vi "from string.vi"(8 "error in":errorcluster, 9 "data":string, 10 "version":string, 11 "TDMS datalogger configuration in":refnum<class "TDMS datalogger configuration.lvclass">) -> (0 "error out":errorcluster, 3 "TDMS datalogger configuration out":refnum<class "TDMS datalogger configuration.lvclass">)   [LabVIEW 2015, in "TDMS datalogger configuration.lvclass"]
doc: "Provides an interface for loading a module configuration from a file or other serialized data source. It is recommended that all children of this class store data in two sets--data required for its own initialization, and any data required for parent initialization--and that each implementation uses the <b>Call Parent Method</b> primitive to de-serialize parent information. As a result, it is expected that every module configuration class calls <b>component configuration.lvclass:From String.vi</b>."
uses:
  TDMS datalogger configuration.lvclass
  <vilib>/NI/Tag Bus Module Framework/channel/TBM channel.lvclass
  <vilib>/NI/LogRotate/options.ctl
  TDMS datalogger configuration.lvclass/TDMS datalogger configuration.ctl
  <vilib>/NI/Tag Bus Module Framework/module configuration/TBM module configuration.lvclass
  <vilib>/NI/Configuration Framework/serializable configuration/NISE_CEF_serializable configuration.lvclass
  <vilib>/NI/LogRotate/LogRotate.lvclass
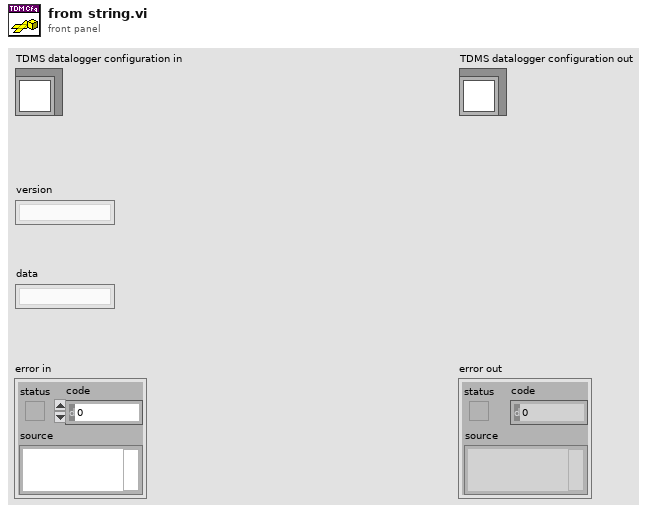
[diagram p1: front panel]
types:
  T1 = cluster{"channel":refnum<class "TBM channel.lvclass">}[]
  T2 = typedef "LogRotate.lvclass/options.ctl" = cluster{"max file size (bytes)":i64, "rotate count":u32, "max age (days)":dbl, "No archive dir":bool, "Archive dir":path}
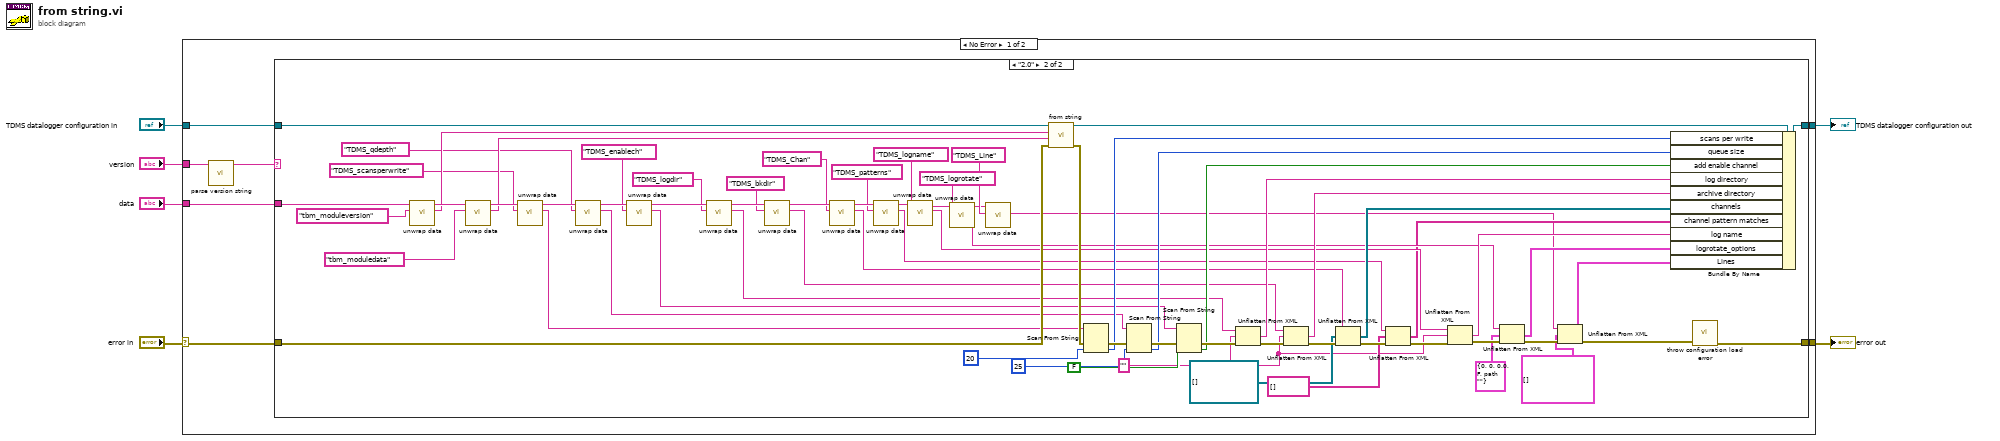
[diagram p0: block diagram]
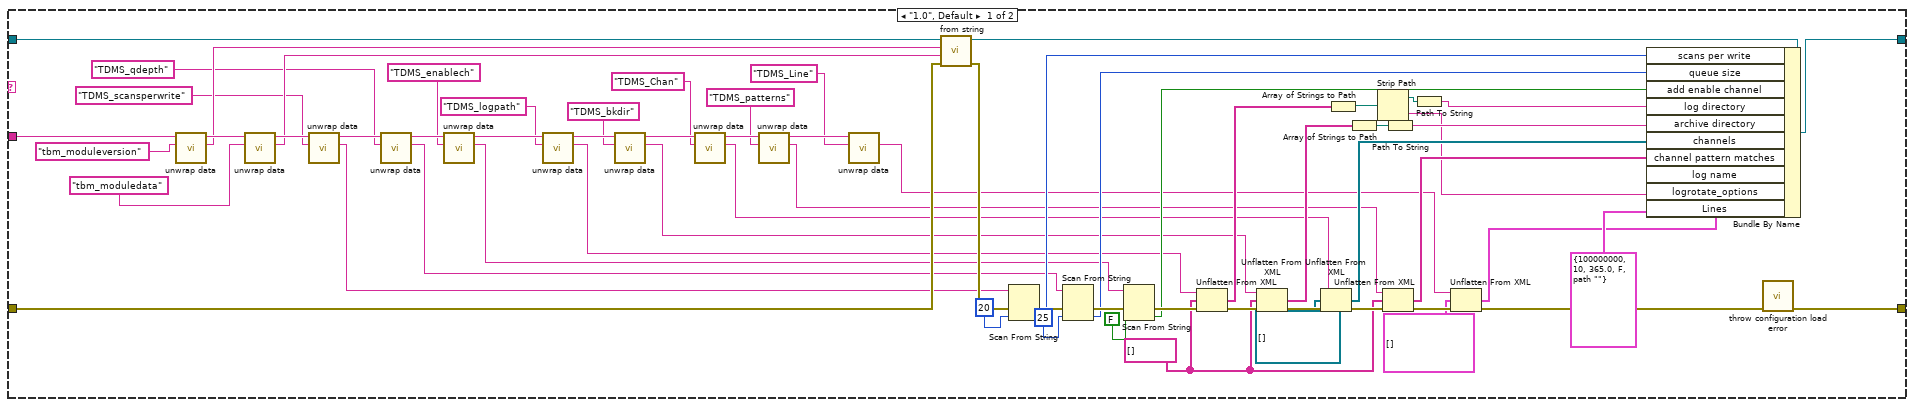
[diagram p2: hidden frame]
diagram:
  n1 = case shown="No Error" "error in" {
    selector: "error in" -> [w7 w150]
    tunnel: "data" -> [w13 _]
    tunnel: "TDMS datalogger configuration in" -> [w12 w149]
    tunnel: [w11 w149] -> w5
    tunnel: [w10 w150] -> w4
    tunnel: "version" -> [w9 _]
    frame No Error {
      n2 = call <vilib>:"parse version string.vi"("full version"=w9) -> ("major.minor version"=w8:string)  [unwired: 7 in, 3 out]
      n3 = case shown="\"2.0\"" w8 {
        tunnel: w13 -> [w61 w131]
        tunnel: w7 -> [w75 w145]
        tunnel: w12 -> [w78 w148]
        tunnel: [w77 w147] -> w11
        tunnel: [w34 w104] -> w10
        frame "1.0", Default {
          w30 = string[] [] ("array of strings")
          n4 = call <vilib>:"unwrap data.vi"("identifier"="tbm_moduleversion" ("additional identifier"), "data to unwrap"=w61) -> ("unwrapped data"=w60:string, "remaining string"=w67:string)  [unwired: 8 in]
          n5 = call <vilib>:"unwrap data.vi"("identifier"="tbm_moduledata" ("additional identifier"), "data to unwrap"=w67) -> ("unwrapped data"=w59:string, "remaining string"=w64:string)  [unwired: 8 in]
          n6 = call <vilib>:"unwrap data.vi"("identifier"="TDMS_scansperwrite" ("additional identifier"), "data to unwrap"=w64) -> ("unwrapped data"=w45:string, "remaining string"=w63:string)  [unwired: 8 in]
          n7 = call <vilib>:"unwrap data.vi"("identifier"="TDMS_qdepth" ("additional identifier"), "data to unwrap"=w63) -> ("unwrapped data"=w43:string, "remaining string"=w62:string)  [unwired: 8 in]
          n8 = call <vilib>:"unwrap data.vi"("identifier"="TDMS_enablech" ("additional identifier"), "data to unwrap"=w62) -> ("unwrapped data"=w41:string, "remaining string"=w49:string)  [unwired: 8 in]
          n9 = call <vilib>:"unwrap data.vi"("identifier"="TDMS_logpath" ("additional identifier"), "data to unwrap"=w49) -> ("unwrapped data"=w39:string, "remaining string"=w48:string)  [unwired: 8 in]
          n10 = call <vilib>:"unwrap data.vi"("identifier"="TDMS_bkdir" ("additional identifier"), "data to unwrap"=w48) -> ("unwrapped data"=w38:string, "remaining string"=w47:string)  [unwired: 8 in]
          n11 = call <vilib>:"unwrap data.vi"("identifier"="TDMS_Chan" ("additional identifier"), "data to unwrap"=w47) -> ("unwrapped data"=w37:string, "remaining string"=w33:string)  [unwired: 8 in]
          n12 = call <vilib>:"unwrap data.vi"("identifier"="TDMS_patterns", "data to unwrap"=w33) -> ("unwrapped data"=w29:string, "remaining string"=w20:string)  [unwired: 8 in]
          n13 = call <vilib>:"unwrap data.vi"("identifier"="TDMS_Line" ("additional identifier"), "data to unwrap"=w20) -> ("unwrapped data"=w15:string)  [unwired: 8 in, 1 out]
          n14 = call-parent "from string.vi"("error in"=w75, "data"=w59, "version"=w60, "module configuration in"=w78) -> ("error out"=w76:errorcluster, "module configuration out"=w74:refnum<class "TDMS datalogger configuration.lvclass">)  [unwired: 6 in]
          n15 = Scan From String(input string=w45, error in=w76, default 1=u16 20 ("scans per write")) -> (error out=w56:errorcluster, output 1=w50:u16)  [unwired: 2 in, 2 out]
          n16 = Scan From String(input string=w43, error in=w56, default 1=u16 25 ("queue size")) -> (error out=w57:errorcluster, output 1=w52:u16)  [unwired: 2 in, 2 out]
          n17 = Scan From String(input string=w41, error in=w57, default 1=FALSE ("add enable channel")) -> (error out=w58:errorcluster, output 1=w54:bool)  [unwired: 2 in, 2 out]
          n18 = Unflatten From XML(xml string=w39, type=w30, error in (no error)=w58) -> (value=w68:string[], error out=w72:errorcluster)
          n19 = Unflatten From XML(xml string=w38, type=w30, error in (no error)=w72) -> (value=w69:string[], error out=w73:errorcluster)
          n20 = Unflatten From XML(xml string=w37, type=refnum<class "TBM channel.lvclass">[] [] ("channels"), error in (no error)=w73) -> (value=w70:refnum<class "TBM channel.lvclass">[], error out=w31:errorcluster)
          n21 = Array of Strings to Path(0:w68) -> (2:w25:path)  [unwired: 1 in]
          n22 = Array of Strings to Path(0:w69) -> (2:w27:path)  [unwired: 1 in]
          n23 = Strip Path(path=w25) -> (stripped path=w23:path, name=w24:string)
          n24 = Unflatten From XML(xml string=w29, type=w30, error in (no error)=w31) -> (value=w28:string[], error out=w18:errorcluster)
          n25 = Path To String(path=w27) -> (string=w26:string)
          n26 = Path To String(path=w23) -> (string=w22:string)
          n27 = Unflatten From XML(xml string=w15, type=T1 [], error in (no error)=w18) -> (value=w14:T1, error out=w17:errorcluster)
          n28 = Bundle By Name(cluster=w74, "scans per write"=w50, "queue size"=w52, "add enable channel"=w54, "log directory"=w22, "archive directory"=w26, "channels"=w70, "channel pattern matches"=w28, "log name"=w24, "logrotate_options"=T2 {"max file size (bytes)"=100000000, "rotate count"=10, "max age (days)"=365.0, "No archive dir"=FALSE, "Archive dir"=path ""}, "Lines"=w14) -> (w77:refnum<class "TDMS datalogger configuration.lvclass">)
          n29 = call <vilib>:"throw configuration load error.vi"("error in"=w17) -> ("error out"=w34:errorcluster)  [unwired: 10 in]
        }
        frame "2.0" {
          w97 = ""
          n30 = call <vilib>:"unwrap data.vi"("identifier"="tbm_moduleversion" ("additional identifier"), "data to unwrap"=w131) -> ("unwrapped data"=w130:string, "remaining string"=w137:string)  [unwired: 8 in]
          n31 = call <vilib>:"unwrap data.vi"("identifier"="tbm_moduledata" ("additional identifier"), "data to unwrap"=w137) -> ("unwrapped data"=w129:string, "remaining string"=w134:string)  [unwired: 8 in]
          n32 = call <vilib>:"unwrap data.vi"("identifier"="TDMS_scansperwrite" ("additional identifier"), "data to unwrap"=w134) -> ("unwrapped data"=w115:string, "remaining string"=w133:string)  [unwired: 8 in]
          n33 = call <vilib>:"unwrap data.vi"("identifier"="TDMS_qdepth" ("additional identifier"), "data to unwrap"=w133) -> ("unwrapped data"=w113:string, "remaining string"=w132:string)  [unwired: 8 in]
          n34 = call <vilib>:"unwrap data.vi"("identifier"="TDMS_enablech" ("additional identifier"), "data to unwrap"=w132) -> ("unwrapped data"=w111:string, "remaining string"=w119:string)  [unwired: 8 in]
          n35 = call <vilib>:"unwrap data.vi"("identifier"="TDMS_logdir" ("additional identifier"), "data to unwrap"=w119) -> ("unwrapped data"=w109:string, "remaining string"=w118:string)  [unwired: 8 in]
          n36 = call <vilib>:"unwrap data.vi"("identifier"="TDMS_bkdir" ("additional identifier"), "data to unwrap"=w118) -> ("unwrapped data"=w108:string, "remaining string"=w117:string)  [unwired: 8 in]
          n37 = call <vilib>:"unwrap data.vi"("identifier"="TDMS_Chan" ("additional identifier"), "data to unwrap"=w117) -> ("unwrapped data"=w107:string, "remaining string"=w103:string)  [unwired: 8 in]
          n38 = call <vilib>:"unwrap data.vi"("identifier"="TDMS_patterns", "data to unwrap"=w103) -> ("unwrapped data"=w99:string, "remaining string"=w95:string)  [unwired: 8 in]
          n39 = call <vilib>:"unwrap data.vi"("identifier"="TDMS_logname", "data to unwrap"=w95) -> ("unwrapped data"=w87:string, "remaining string"=w93:string)  [unwired: 8 in]
          n40 = call <vilib>:"unwrap data.vi"("identifier"="TDMS_logrotate", "data to unwrap"=w93) -> ("unwrapped data"=w90:string, "remaining string"=w84:string)  [unwired: 8 in]
          n41 = call <vilib>:"unwrap data.vi"("identifier"="TDMS_Line" ("additional identifier"), "data to unwrap"=w84) -> ("unwrapped data"=w80:string)  [unwired: 8 in, 1 out]
          n42 = call-parent "from string.vi"("error in"=w145, "data"=w129, "version"=w130, "module configuration in"=w148) -> ("error out"=w146:errorcluster, "module configuration out"=w144:refnum<class "TDMS datalogger configuration.lvclass">)  [unwired: 6 in]
          n43 = Scan From String(input string=w115, error in=w146, default 1=u16 20 ("scans per write")) -> (error out=w126:errorcluster, output 1=w120:u16)  [unwired: 2 in, 2 out]
          n44 = Scan From String(input string=w113, error in=w126, default 1=u16 25 ("queue size")) -> (error out=w127:errorcluster, output 1=w122:u16)  [unwired: 2 in, 2 out]
          n45 = Scan From String(input string=w111, error in=w127, default 1=FALSE ("add enable channel")) -> (error out=w128:errorcluster, output 1=w124:bool)  [unwired: 2 in, 2 out]
          n46 = Unflatten From XML(xml string=w109, type=w97, error in (no error)=w128) -> (value=w138:string, error out=w142:errorcluster)
          n47 = Unflatten From XML(xml string=w108, type=w97, error in (no error)=w142) -> (value=w139:string, error out=w143:errorcluster)
          n48 = Unflatten From XML(xml string=w107, type=refnum<class "TBM channel.lvclass">[] [] ("channels"), error in (no error)=w143) -> (value=w140:refnum<class "TBM channel.lvclass">[], error out=w101:errorcluster)
          n49 = Unflatten From XML(xml string=w99, type=string[] [] ("array of strings"), error in (no error)=w101) -> (value=w86:string[], error out=w98:errorcluster)
          n50 = Unflatten From XML(xml string=w87, type=w97, error in (no error)=w98) -> (value=w96:string, error out=w91:errorcluster)
          n51 = Unflatten From XML(xml string=w90, type=T2 {"max file size (bytes)"=0, "rotate count"=0, "max age (days)"=0.0, "No archive dir"=FALSE, "Archive dir"=path ""} ("logrotate_options"), error in (no error)=w91) -> (value=w88:T2, error out=w83:errorcluster)
          n52 = Unflatten From XML(xml string=w80, type=T1 [], error in (no error)=w83) -> (value=w79:T1, error out=w82:errorcluster)
          n53 = Bundle By Name(cluster=w144, "scans per write"=w120, "queue size"=w122, "add enable channel"=w124, "log directory"=w138, "archive directory"=w139, "channels"=w140, "channel pattern matches"=w86, "log name"=w96, "logrotate_options"=w88, "Lines"=w79) -> (w147:refnum<class "TDMS datalogger configuration.lvclass">)
          n54 = call <vilib>:"throw configuration load error.vi"("error in"=w82) -> ("error out"=w104:errorcluster)  [unwired: 10 in]
        }
      }
    }
    frame Error {
    }
  }
  "error out" <- w4
  "TDMS datalogger configuration out" <- w5
